vi "getThrust.vi"(8 "error in (no error)":errorcluster, 10 "Throttle % [0-100]":dbl, 11 "Scale Emulator in":refnum<class "Scale Emulator.lvclass">) -> (0 "error out":errorcluster, 2 "Thrust [g]":dbl, 3 "Scale Emulator out":refnum<class "Scale Emulator.lvclass">)   [LabVIEW 2015, in "Scale Emulator.lvclass"]
uses:
  Scale Emulator.lvclass
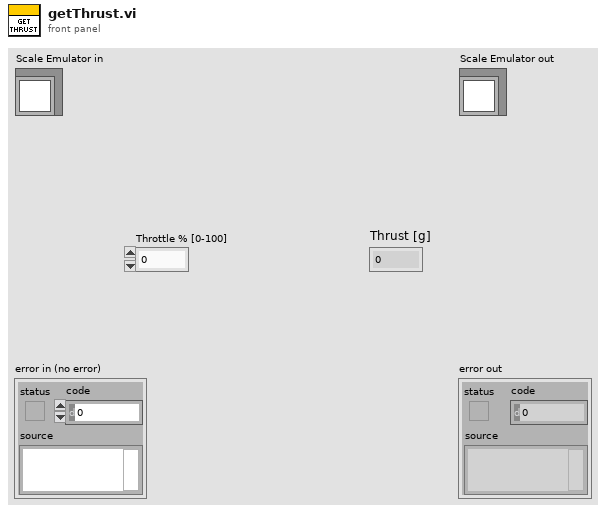
[diagram p1: front panel]
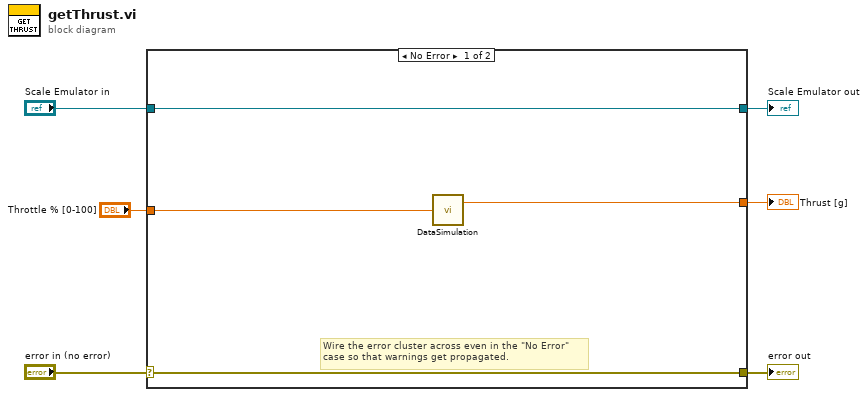
[diagram p0: block diagram]
diagram:
  n1 = case shown="No Error" "error in (no error)" {
    selector: "error in (no error)" -> [w9 w12]
    tunnel: [w9 w12] -> w5
    tunnel: [w10 w11] -> w3
    tunnel: "Scale Emulator in" -> [w10 w11]
    tunnel: [w8 _] -> w2
    tunnel: "Throttle % [0-100]" -> [w7 _]
    frame No Error {
      # "Wire the error cluster across even in the \"No Error\"\ncase so that warnings get propagated."
      n2 = call "DataSimulation.vi"("Throttle % [0-100]"=w7) -> ("Thrust from Force Gauge"=w8:dbl)  [unwired: 2 in, 1 out]
    }
    frame Error {
    }
  }
  "error out" <- w5
  "Scale Emulator out" <- w3
  "Thrust [g]" <- w2
